vi "testGetValFromVariant.vi"(8 "error in (no error)":errorcluster) -> (0 "error out":errorcluster)   [LabVIEW 2018]
uses:
  src/VariantTool/getValFromVariant_string.vi
  <vilib>/addons/_JKI Toolkits/Caraya/classes/Assert/Assert Equal Value and Type_Variant.vi
  src/VariantTool/getValFromVariant_double.vi
  src/VariantTool/getValFromVariant_I32.vi
  src/VariantTool/getValFromVariant_enum.vi
  <vilib>/addons/_JKI Toolkits/Caraya/classes/Test/Test.lvclass
  <vilib>/addons/_JKI Toolkits/Caraya/classes/Assert/Assert.lvclass
panel:
  in  "Enum":enum16{"", "enum1", "enum2"}(ring)
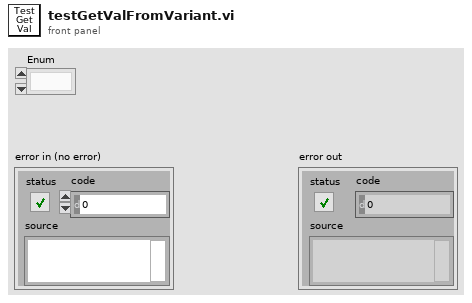
[diagram p1: front panel]
types:
  T1 = cluster{"nameI32":i32, "nameDouble":dbl, "nameString":string, "nameEnum":enum16{"", "enum1", "enum2"}}
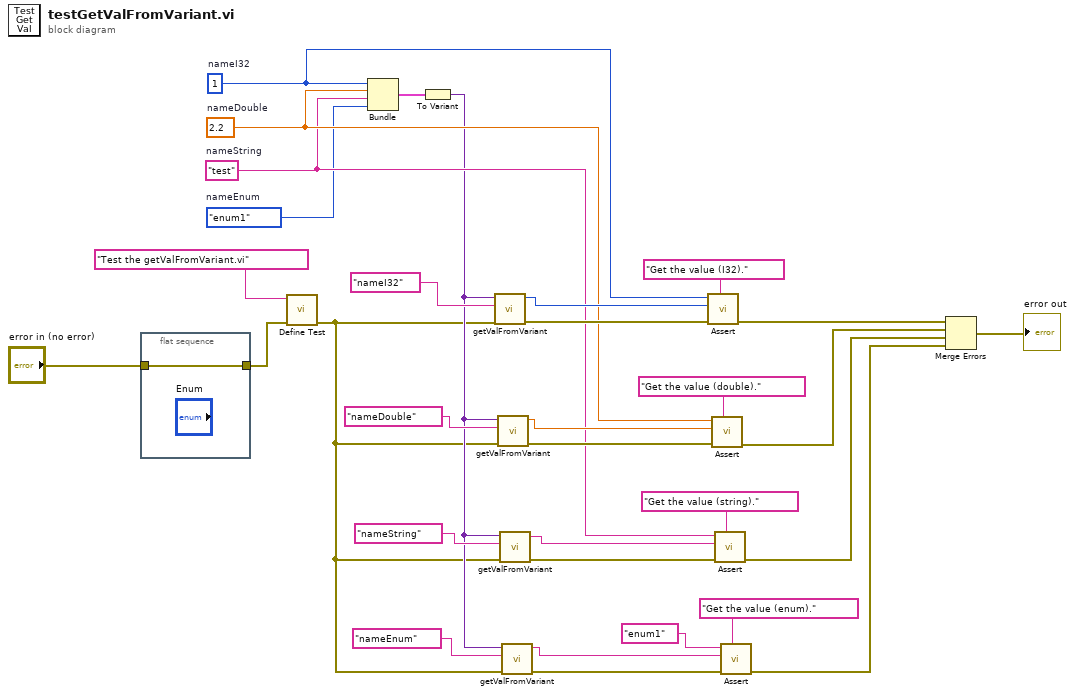
[diagram p0: block diagram]
diagram:
  w11 = enum16{"", "enum1", "enum2"}."enum1"  # nameEnum
  w13 = "test"  # nameString
  w25 = 2.2  # nameDouble
  w28 = 1  # nameI32
  n1 = flat-sequence {
    tunnel: [w33] -> w6
    tunnel: "error in (no error)" -> [w33]
    frame #0 {
    }
  }
  n2 = call <vilib>:"Define Test.vi"("error in (no error)"=w6, "Label (VI Title)"="Test the getValFromVariant.vi") -> ("error out"=w9:errorcluster)  [unwired: 9 in]
  n3 = Bundle("nameI32"=w28, "nameDouble"=w25, "nameString"=w13, "nameEnum"=w11) -> (w31:T1)  [unwired: 1 in]
  n4 = To Variant(anything=w31) -> (Variant=w10:variant)
  n5 = call-poly "getValFromVariant.vi"("error in (no error)"=w9, "name"="nameI32", "variant"=w10) -> ("error out"=w26:errorcluster, "value"=w27:i32)  [unwired: 7 in]
  n6 = call-poly "getValFromVariant.vi"("error in (no error)"=w9, "name"="nameDouble", "variant"=w10) -> ("error out"=w23:errorcluster, "value"=w24:dbl)  [unwired: 7 in]
  n7 = call-poly "getValFromVariant.vi"("error in (no error)"=w9, "name"="nameString", "variant"=w10) -> ("error out"=w15:errorcluster, "value"=w14:string)  [unwired: 7 in]
  n8 = call-poly "getValFromVariant.vi"("error in (no error)"=w9, "name"="nameEnum", "variant"=w10) -> ("error out"=w5:errorcluster, "value"=w4:string)  [unwired: 7 in]
  n9 = call-poly <vilib>:"Assert.vi"("Label"="Get the value (I32).", "error in (no error)"=w26, "Y"=w27, "X"=w28) -> ("error out"=w22:errorcluster)  [unwired: 7 in]
  n10 = call-poly <vilib>:"Assert.vi"("Label"="Get the value (double).", "error in (no error)"=w23, "Y"=w24, "X"=w25) -> ("error out"=w21:errorcluster)  [unwired: 7 in]
  n11 = call-poly <vilib>:"Assert.vi"("Label"="Get the value (string).", "error in (no error)"=w15, "Y"=w14, "X"=w13) -> ("error out"=w12:errorcluster)  [unwired: 7 in]
  n12 = call-poly <vilib>:"Assert.vi"("Label"="Get the value (enum).", "error in (no error)"=w5, "Y"=w4, "X"="enum1") -> ("error out"=w2:errorcluster)  [unwired: 7 in]
  n13 = Merge Errors(w22, w21, w12, w2) -> (→"error out":errorcluster)
